vi "Register gRPC Server.vi"(8 "error in (no error)":errorcluster, 10 "gRPC ID":T1, 11 "CIFLauncher in":refnum<class "CIFPluginLoader.lvclass">) -> (0 "error out":errorcluster, 3 "CIFLauncher out":refnum<class "CIFPluginLoader.lvclass">)   [LabVIEW 2021, in "CIFPluginLoader.lvclass"]
uses:
  CIFPluginLoader.lvclass
  <vilib>/gRPC/LabVIEW gRPC Library/Shared/grpcId.ctl
  CIF_PluginLoader_server/RPC Service/PluginLoader/PluginLoader.lvclass
  C:/Program Files/National Instruments/LabVIEW 2021/vi.lib/gRPC/LabVIEW gRPC Servicer/ServiceBase/ServiceBase.lvclass
  <vilib>/gRPC/LabVIEW gRPC Library/Server API/Server/Register Message Metadata.vi
  <vilib>/gRPC/LabVIEW gRPC Library/Server API/Server/Register Enum Metadata.vi
  CIFPluginLoader.lvclass/CIFPluginLoader.ctl
  CIF_PluginLoader_server/CIF_PluginLoader_server.lvlib
  <vilib>/gRPC/LabVIEW gRPC Library/grpc-lvsupport-release.lvlib
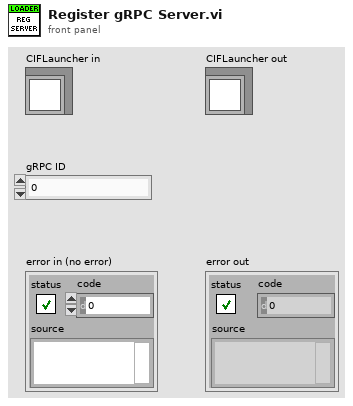
[diagram p1: front panel]
types:
  T1 = typedef "grpc-lvsupport-release.lvlib/grpcId.ctl" = u64
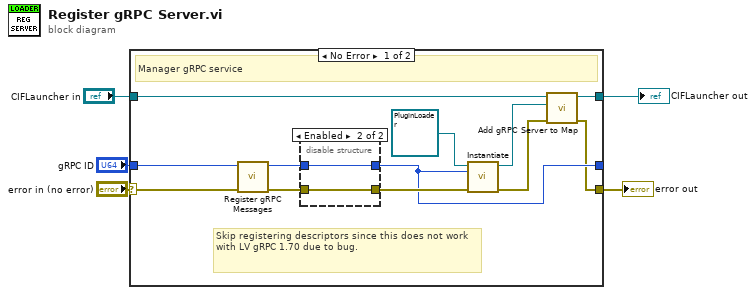
[diagram p0: block diagram]
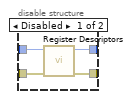
[diagram p2: hidden frame]
diagram:
  n1 = case shown="No Error" "error in (no error)" {
    selector: "error in (no error)" -> [w15 w26]
    tunnel: [w6 w26] -> w4
    tunnel: [w11 w25] -> w1
    tunnel: "CIFLauncher in" -> [w12 w25]
    tunnel: "gRPC ID" -> [w14 w24]
    tunnel: [w7 w24] -> _
    frame No Error {
      # "Skip registering descriptors since this does not work with LV gRPC 1.70 due to bug."
      # "Manager gRPC service"
      n2 = call "Register gRPC Messages.vi"("error in (no error)"=w15, "gRPC ID"=w14) -> ("error out"=w16:errorcluster, "gRPC ID Out"=w17:T1)  [unwired: 8 in]
      n3 = disable-structure shown="Enabled" {
        disable-tunnel: w17 -> [w21 w23]
        disable-tunnel: w16 -> [w20 w22]
        disable-tunnel: [w19 w22] -> w13
        disable-tunnel: [w18 w23] -> w7
        frame Disabled {
          n4 = call "Register Descriptors.vi"("error in (no error)"=w20, "gRPC ID"=w21) -> ("error out"=w19:errorcluster, "gRPC ID Out"=w18:T1)  [unwired: 8 in]
        }
        frame Enabled {
        }
      }
      n5 = call-dynamic "Instantiate.vi"("error in"=w13, "gRPCid"=w7, "gRPC service in"=refnum<class "PluginLoader.lvclass"> refnum ("CIF_Plugin_Core_server.lvlib:PluginCore.lvclass")) -> ("error out"=w9:errorcluster, "gRPC service out"=w8:refnum<class "PluginLoader.lvclass">)  [unwired: 7 in]
      n6 = call "Add gRPC Server to Map.vi"("error in (no error)"=w9, "gRPC Server Class"=w8, "CIFLauncher in"=w12) -> ("error out"=w6:errorcluster, "CIFLauncher out"=w11:refnum<class "CIFPluginLoader.lvclass">)  [unwired: 7 in]
    }
    frame Error {
    }
  }
  "error out" <- w4
  "CIFLauncher out" <- w1
